vi "XMLExtractTableHeader.vi"(11 "XMLIn":string) -> (3 "TableHeaderInfo":string)   [LabVIEW 2014]
uses:
  <vilib>/regexp/Match Regular Expression.xnode
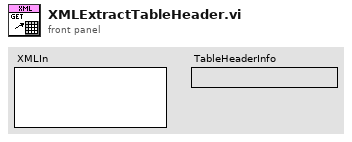
[diagram p1: front panel]
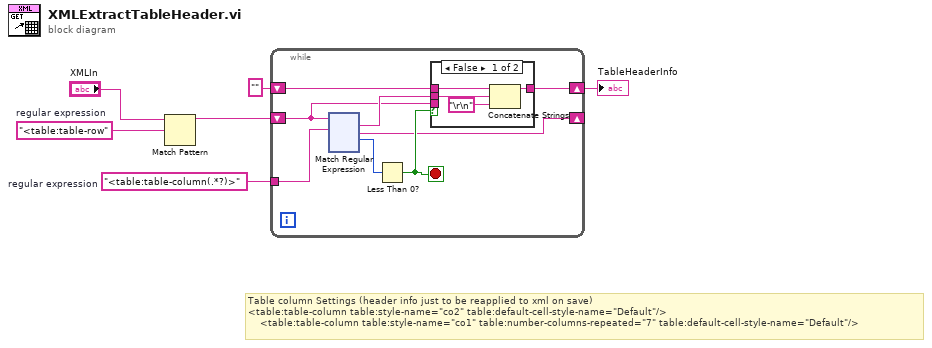
[diagram p0: block diagram]
diagram:
  w4 = "<table:table-column(.*?)>"  # regular expression
  w2 = "<table:table-row"  # regular expression
  # "Table column Settings (header info just to be reapplied to xml on save)\n<table:table-column table:style-name=\"co2\" table:default-cell-style-name=\"Default\"/>\n\t\t\t\t<table:table-column table:style-name=\"co1\" table:number-columns-repeated=\"7\" table:default-cell-style-name=\"Default\"/>"
  n1 = Match Pattern(string="XMLIn", regular expression=w2) -> (before substring=w3:string)  [unwired: 1 in, 3 out]
  n2 = while {
    shift-right: [w7] -> _
    shift-left: w3 -> [w8]
    tunnel: w4 -> [w14]
    shift-right: [w11] -> w6
    shift-left: "" -> [w13]
    stop <- w9 stop-if-true
    n3 = xnode "Match Regular Expression"("input string"=w8, "regular expression"=w14) -> ("whole match"=w12:string, "after match"=w7:string, "offset past match"=w10:i32)  [unwired: 4 in, 2 out]
    n4 = Less Than 0?(x=w10) -> (x < 0?=w9:bool)
    n5 = case shown="False" w9 {
      tunnel: w13 -> [w18 w19]
      tunnel: w12 -> [w17 _]
      tunnel: [w16 w19] -> w11
      tunnel: w8 -> [_ _]
      frame False {
        n6 = Concatenate Strings(w18, w17, "\r\n") -> (w16:string)
      }
      frame True {
      }
    }
  }
  "TableHeaderInfo" <- w6
